vi "Generate PCB coverage.vi"(0 "Inspection Data":T2, 5 "error in (no error)":errorcluster) -> (12 "DataOut":T1, 19 "error out":errorcluster)   [LabVIEW 2013, in "Manipulate IPF.lvlib"]
uses:
  Manipulate IPF.lvlib
  3013/code/Modules/GUI/GUI_5/subPanels/edit/type_def/data.ctl
  3013/code/Modules/Configuration/type_def/Scan Params.ctl
  3013/code/Modules/Configuration/type_def/Profile Resolution.ctl
  3013/code/Modules/Preprocess Data/type_def/direction.ctl
  3013/code/Modules/Inspection/Data/Panel_class/type_def/Config File data.ctl
  3013/code/Modules/Inspection/type_def/Pos and Rot.ctl
  3013/code/Modules/Inspection/Data/PCB_class/type_def/PCB Params.ctl
  3013/code/Modules/Inspection/Data/Panel_class/type_def/BarCode Params.ctl
  3013/code/Modules/Barcode Reader/type_def/id.ctl
  3013/code/Modules/Inspection/Data/Panel_class/type_def/inspection data.ctl
  3013/code/Modules/Inspection/type_def/Range Limits.ctl
  <userlib>/_OpenG.lib/file/file.llb/File Exists - Scalar__ogtk.vi
  <vilib>/Utility/file.llb/Read From Spreadsheet File (string).vi
  <userlib>/_OpenG.lib/file/file.llb/Convert File Extension (String)__ogtk.vi
  <vilib>/Utility/file.llb/Write To Spreadsheet File (string).vi
  <userlib>/_OpenG.lib/string/string.llb/Trim Whitespace (String)__ogtk.vi
  <vilib>/Utility/file.llb/Read From Spreadsheet File (DBL).vi
  Mike/APG_mike a3Di.lvlib
  3D Viewer/3D Viewer.lvlib
  <vilib>/Analysis/geometry.llb/Point in Polygon Position.ctl
  <vilib>/Analysis/NI_AAL_Geometry.lvlib
  <vilib>/Analysis/geometry.llb/Point in Polygon (Array).vi
  3013/code/subVIs/Library/array/AmFax Array.lvlib
  3013/code/Modules/Inspection/Inspection.lvlib
  3013/code/Modules/Inspection/Data/PCB_class/PCB.lvclass
  3013/code/Modules/Barcode Reader/Barcode Reader.lvlib
  3013/code/Modules/Inspection/Data/Panel_class/Panel.lvclass
  3013/code/Modules/Configuration/Config.lvlib
  3013/code/Modules/Preprocess Data/PreProcess.lvlib
  3013/code/Modules/GUI/GUI_5/subPanels/edit/edit.lvlib
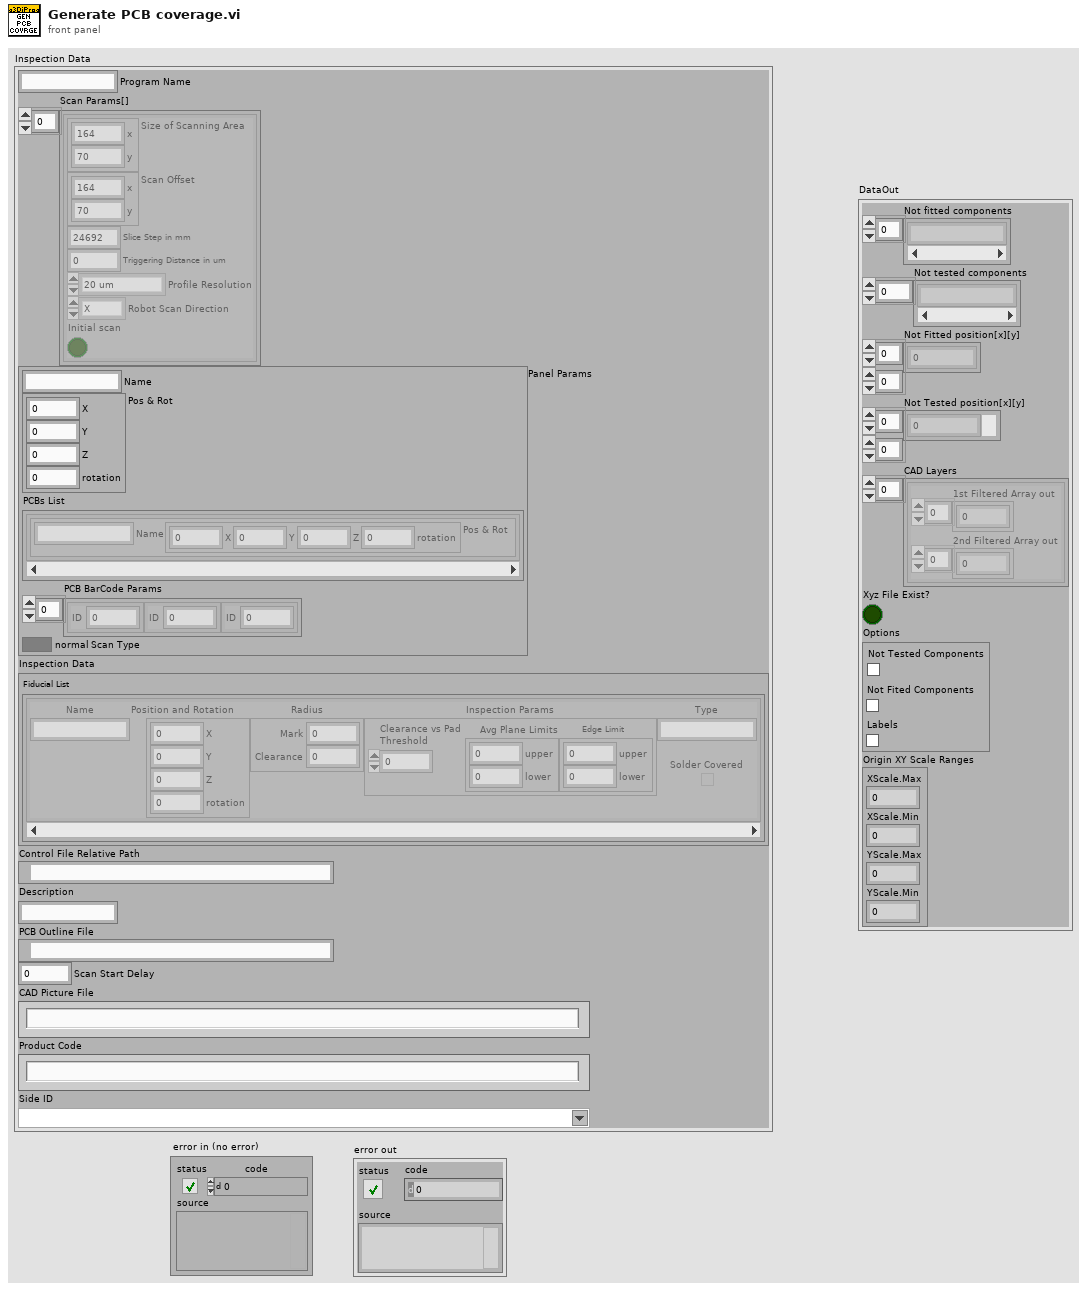
[diagram p1: front panel]
types:
  T1 = cluster{"Not fitted components":string[], "Not tested components":string[], "Not Fitted position[x][y] ":dbl[][], "Not Tested position[x][y]":dbl[][], "CAD Layers":cluster{"1st Filtered Array out":sgl[], "2nd Filtered Array out":sgl[]}[], "Xyz File Exist? ":bool, "Options":cluster{"Enable Not Tested Components":bool, "Enable Not Fited Components":bool, "Enable Labels":bool}, "Origin XY Scale Ranges":cluster{"XScale.Max":dbl, "XScale.Min":dbl, "YScale.Max":dbl, "YScale.Min":dbl}}
  T2 = typedef "GUI.lvlib/subPanel.lvlib/edit.lvlib/data.ctl" = cluster{"Program Name":string, "Scan Params[]":T3[], "Panel Params":T6, "Inspection Data":T11, "Control File Relative Path":path, "Description":string, "PCB Outline File":path, "Scan Start Delay":dbl, "CAD Picture File":string, "Product Code":string, "Side ID":string}
  T3 = typedef "Config.lvlib/Scan Params.ctl" = cluster{"Size of Scanning Area":cluster{"x":dbl, "y":dbl}, "Scan Offset":cluster{"x":dbl, "y":dbl}, "Slice Step in mm":dbl, "Triggering Distance in mm":dbl, "Triggering Distance in um":dbl, "Profile Resolution":T4, "Version":string, "Robot Scan Direction":T5, "Initial scan":bool}
  T4 = typedef "Config.lvlib/Profile Resolution.ctl" = enum8{"20 um", "40 um"}
  T5 = typedef "PreProcess.lvlib/direction.ctl" = enum8{"X", "Y"}
  T6 = typedef "Inspection.lvlib/Panel.lvclass/Config File data.ctl" = cluster{"Name":string, "Pos & Rot":T7, "PCBs List":cluster{"PCB Params":T8}[], "PCB BarCode Params":T9[], "Scan Type":bool}
  T7 = typedef "Inspection.lvlib/Pos and Rot.ctl" = cluster{"X":dbl, "Y":dbl, "Z":dbl, "rotation":dbl}
  T8 = typedef "Inspection.lvlib/PCB.lvclass/PCB Params.ctl" = cluster{"Name":string, "Pos & Rot":T7}
  T9 = typedef "Inspection.lvlib/Panel.lvclass/BarCode Params.ctl" = cluster{"ID":T10}
  T10 = typedef "Barcode Reader.lvlib/id.ctl" = u8
  T11 = typedef "Inspection.lvlib/Panel.lvclass/inspection data.ctl" = cluster{"Fiducial List":cluster{"Name":string, "Position and Rotation":T7, "Radius":cluster{"Mark":dbl, "Clearance":dbl}, "Inspection Params":cluster{"Clearance vs Pad\nThreshold":dbl, "Avg Plane Limits":T12, "Edge Limit":T12}, "Type":string, "Solder Covered":bool}[]}
  T12 = typedef "Inspection.lvlib/Range Limits.ctl" = cluster{"upper":sgl, "lower":sgl}
  T13 = cluster{"ODB2CPF.exe":path, "TCFToArtworkCPF.exe":path, "TCFToCPFLabels.exe":path, "7z.exe":path, "UpdateTCFLibrary.exe":path, "a3DiPackageTests":path, "Error Codes":path, "TCFToCuboidRefCPF":path, "TCFToArtworkRefCPF":path, "ExtractPKG":path, "ExtractTCFFromODBFileForPKG":path, "OutLineFilterTCFPKG":path, "GenerateLibraryFromTCF":path, "FlipCPF":path, "FlipTCF":path, "TCFToJointBridgeCPF":path, "TCFToJointFR4CPF":path, "UpdateTCFPartNoFrCompName":path}
  T14 = typedef "NI_AAL_Geometry.lvlib/Point in Polygon Position.ctl" = u16
  T15 = cluster{"1st Filtered Array out":sgl[], "2nd Filtered Array out":sgl[]}
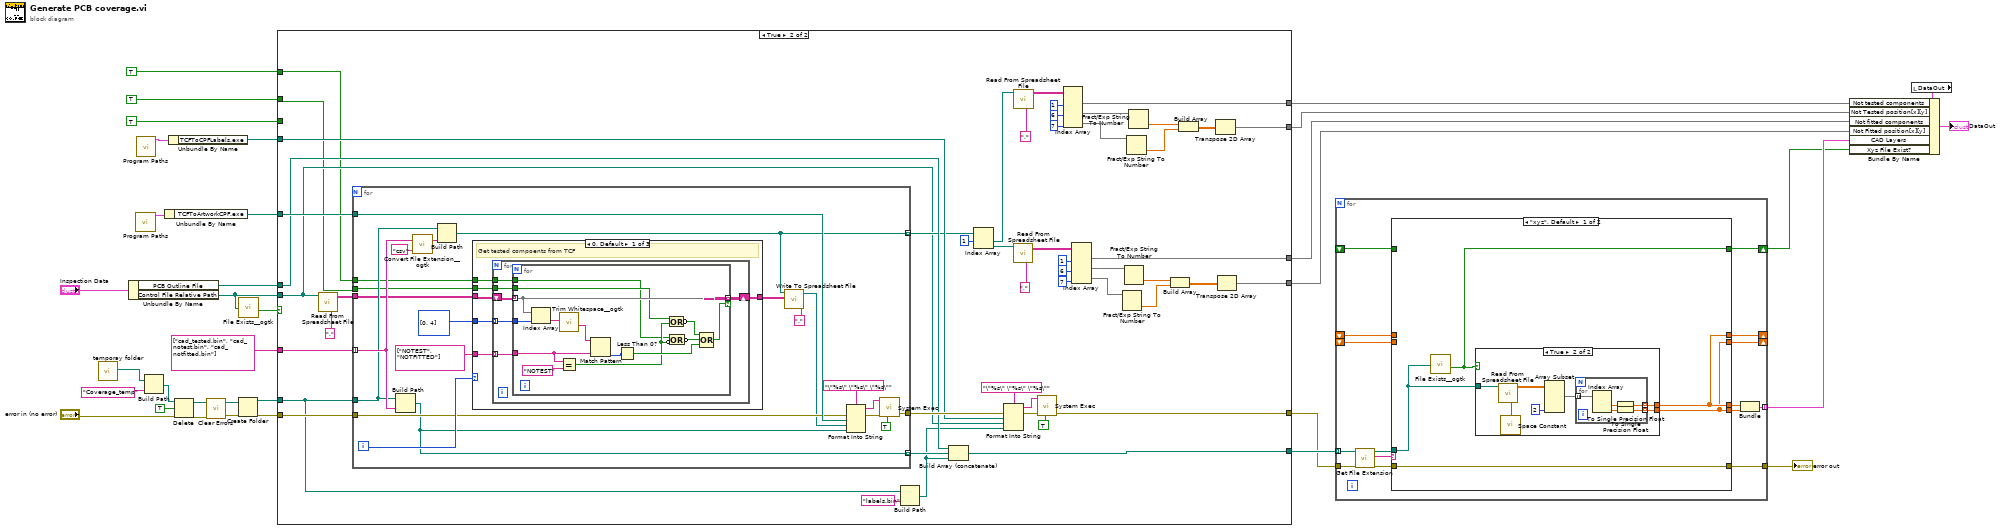
[diagram p0: block diagram]
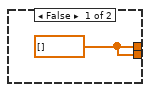
[diagram p2: hidden frame]
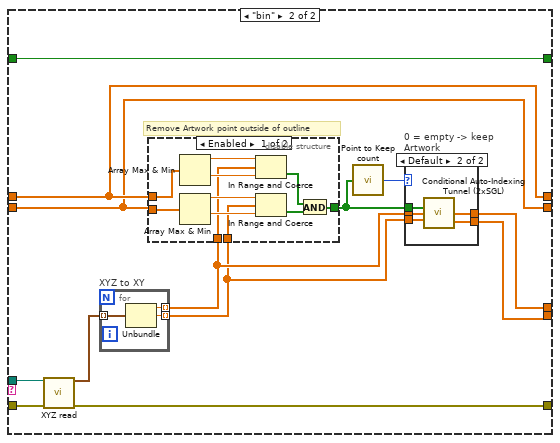
[diagram p3: hidden frame]
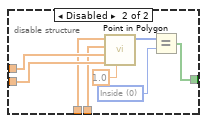
[diagram p5: hidden frame]
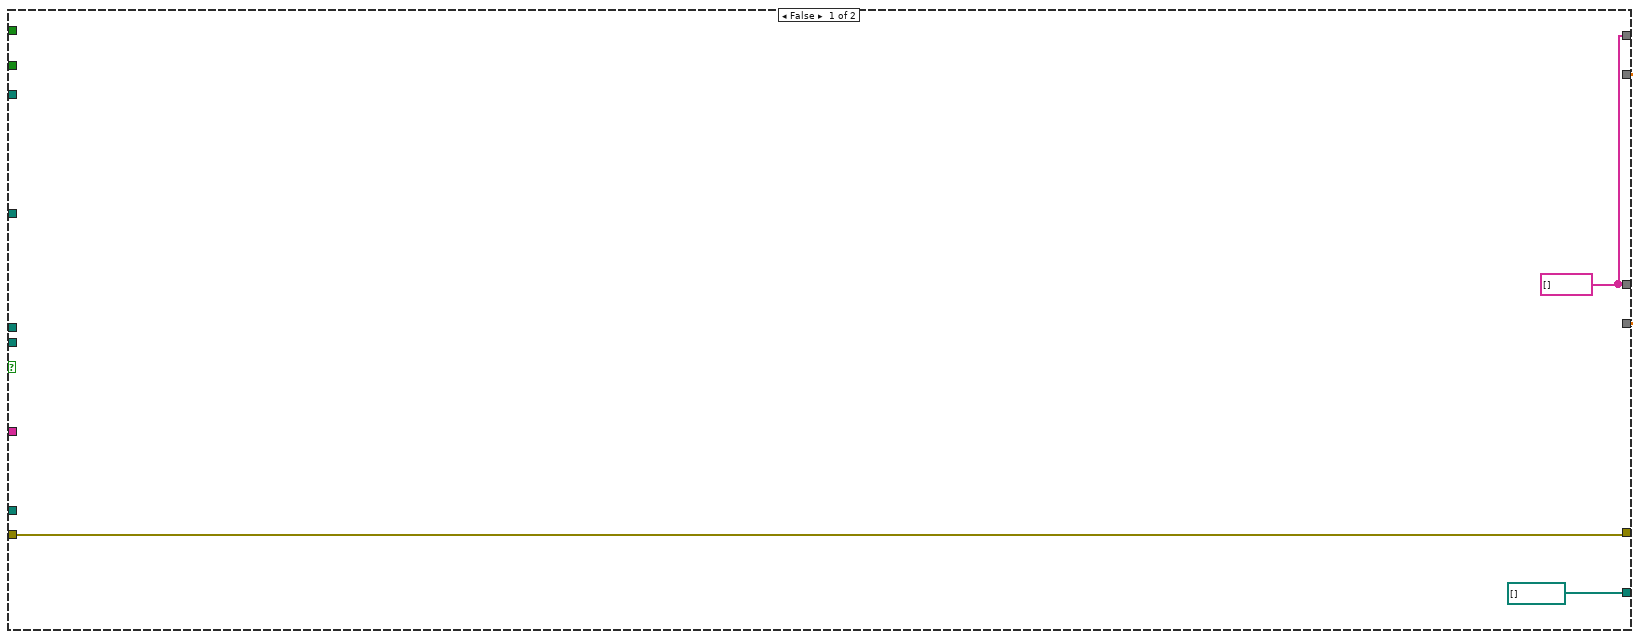
[diagram p6: hidden frame]
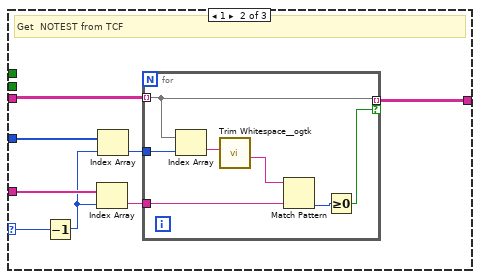
[diagram p7: hidden frame]
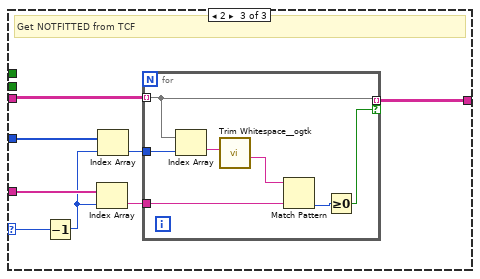
[diagram p8: hidden frame]
diagram:
  n1 = call "temporay folder.vi"() -> ("temporay folder"=w33:path)  [unwired: 11 in]
  n2 = Unbundle By Name("Inspection Data") -> ("PCB Outline File"=w15:path, "Control File Relative Path"=w17:path)
  n3 = call "Program Paths.vi"() -> ("Program paths"=w31:T13)  [unwired: 10 in]
  n4 = call "Program Paths.vi"() -> ("Program paths"=w21:T13)  [unwired: 10 in]
  n5 = Build Path(base path=w33, name or relative path="Coverage_temp") -> (appended path=w27:path)
  n6 = Unbundle By Name(w31) -> ("TCFToArtworkCPF.exe"=w28:path)
  n7 = Unbundle By Name(w21) -> ("TCFToCPFLabels.exe"=w20:path)
  n8 = Delete(path (use dialog)=w27, entire hierarchy (F)=TRUE, error in="error in (no error)") -> (deleted path=w23:path, error out=w25:errorcluster)  [unwired: 2 in, 1 out]
  n9 = call <vilib>:"Clear Errors.vi"("error in (no error)"=w25) -> ("error out"=w24:errorcluster)  [unwired: 6 in]
  n10 = Create Folder(path (use dialog)=w23, error in=w24) -> (created path=w19:path, error out=w22:errorcluster)  [unwired: 1 in, 1 out]
  n11 = call-poly <userlib>:"File Exists__ogtk.vi"("file path"=w17) -> ("exists"=w16:bool)  [unwired: 6 in, 1 out]
  n12 = case shown="True" w16 {
    tunnel: string[] ["cad_tested.bin", "cad_notest.bin", "cad_notfitted.bin"] -> [_ w87]
    tunnel: w28 -> [_ w86]
    tunnel: w22 -> [w38 w85]
    tunnel: [w38 w83] -> w2
    tunnel: w20 -> [_ w82]
    tunnel: w19 -> [_ w81]
    tunnel: w17 -> [_ w48]
    tunnel: w15 -> [_ w78]
    tunnel: [w37 w70] -> w11
    tunnel: [w37 w62] -> w14
    tunnel: [dbl[][] [] w50] -> w9
    tunnel: [dbl[][] [] w52] -> w10
    tunnel: TRUE ("Not Fited Components") -> [_ w46]
    tunnel: TRUE ("Not Tested Components") -> [_ w45]
    tunnel: TRUE ("Labels") -> [_ _]
    tunnel: [path[] [] w44] -> w5
    frame False {
      w37 = string[] [] ("all rows")
    }
    frame True {
      n13 = call-poly <vilib>:"Read From Spreadsheet File.vi"("delimiter (\\t)"="," ("delimiter (\\t)"), "file path (dialog if empty)"=w48) -> ("all rows"=w47:string[][])  [unwired: 5 in, 4 out]
      n14 = for {
        tunnel: w87 -> [w103] mode=indexing
        tunnel: w85 -> [w99]
        tunnel: w81 -> [w102]
        tunnel: w86 -> [w101]
        tunnel: [w98] -> w84
        tunnel: [w88] -> w79 mode=indexing
        tunnel: [w92] -> w77 mode=indexing
        tunnel: w47 -> [w91]
        tunnel: w46 -> [w90]
        tunnel: w45 -> [w89]
        i -> [w100]
        n15 = Build Path(base path=w102, name or relative path=w103) -> (appended path=w88:path)
        n16 = call-poly <userlib>:"Convert File Extension__ogtk.vi"("new ending (none)"="csv", "file name"=w103) -> ("new filename"=w109:string)  [unwired: 1 out]
        n17 = Build Path(base path=w102, name or relative path=w109) -> (appended path=w92:path)
        n18 = case shown="0, Default" w100 {
          selector: w100 -> [_ w143 w158]
          tunnel: w91 -> [w115 w142 w157]
          tunnel: [w114 w141 w156] -> w95
          tunnel: i32[] [0, 4] -> [w113 w140 w155]
          tunnel: string[] ["NOTEST", "NOTFITTED"] -> [w112 w139 w154]
          tunnel: w90 -> [w110 _ _]
          tunnel: w89 -> [w111 _ _]
          frame 0, Default {
            # "Get tested compoents from TCF"
            n19 = for {
              tunnel: w113 -> [w119] mode=indexing
              tunnel: w112 -> [w120] mode=indexing
              shift-right: [w121] -> w114
              shift-left: w115 -> [w118]
              tunnel: w111 -> [w116]
              tunnel: w110 -> [w117]
              n20 = for {
                tunnel: w118 -> [w135] mode=indexing
                tunnel: [w135] -> w121 mode=indexing if=w130
                tunnel: w120 -> [w128]
                tunnel: w119 -> [w131]
                tunnel: w117 -> [w123]
                tunnel: w116 -> [w122]
                n21 = Index Array(array=w135, index=w131) -> (element=w134:string)
                n22 = call-poly <userlib>:"Trim Whitespace__ogtk.vi"("String in"=w134) -> ("String out"=w133:string)  [unwired: 6 in]
                n23 = Equal?(x=w128, y="NOTEST") -> (x = y?=w125:bool)
                n24 = Match Pattern(string=w133, regular expression=w128) -> (offset past match=w132:i32)  [unwired: 1 in, 3 out]
                n25 = Less Than 0?(x=w132) -> (x < 0?=w126:bool)
                n26 = Compound Arithmetic op=OR(w123, w125) -> (invert w124:bool)
                n27 = Compound Arithmetic op=OR(w122, invert w125) -> (invert w129:bool)
                n28 = Compound Arithmetic op=OR(w124, w129, w126) -> (w130:bool)
              }
            }
          }
          frame 1 {
            # "Get  NOTEST from TCF"
            n29 = Decrement(x=w143) -> (x-1=w136:i32)
            n30 = Index Array(array=w139, index=w136) -> (element=w138:string)
            n31 = Index Array(array=w140, index=w136) -> (element=w137:i32)
            n32 = for {
              tunnel: w142 -> [w150] mode=indexing
              tunnel: [w150] -> w141 mode=indexing if=w146
              tunnel: w138 -> [w145]
              tunnel: w137 -> [w144]
              n33 = Index Array(array=w150, index=w144) -> (element=w149:string)
              n34 = call-poly <userlib>:"Trim Whitespace__ogtk.vi"("String in"=w149) -> ("String out"=w148:string)  [unwired: 6 in]
              n35 = Match Pattern(string=w148, regular expression=w145) -> (offset past match=w147:i32)  [unwired: 1 in, 3 out]
              n36 = Greater Or Equal To 0?(x=w147) -> (x >= 0?=w146:bool)
            }
          }
          frame 2 {
            # "Get NOTFITTED from TCF"
            n37 = Decrement(x=w158) -> (x-1=w151:i32)
            n38 = Index Array(array=w154, index=w151) -> (element=w153:string)
            n39 = Index Array(array=w155, index=w151) -> (element=w152:i32)
            n40 = for {
              tunnel: w157 -> [w165] mode=indexing
              tunnel: [w165] -> w156 mode=indexing if=w161
              tunnel: w153 -> [w160]
              tunnel: w152 -> [w159]
              n41 = Index Array(array=w165, index=w159) -> (element=w164:string)
              n42 = call-poly <userlib>:"Trim Whitespace__ogtk.vi"("String in"=w164) -> ("String out"=w163:string)  [unwired: 6 in]
              n43 = Match Pattern(string=w163, regular expression=w160) -> (offset past match=w162:i32)  [unwired: 1 in, 3 out]
              n44 = Greater Or Equal To 0?(x=w162) -> (x >= 0?=w161:bool)
            }
          }
        }
        n45 = call-poly <vilib>:"Write To Spreadsheet File.vi"("delimiter (\\t)"="," ("delimiter (\\t)"), "2D data"=w95, "file path (dialog if empty)"=w92) -> ("new file path (Not A Path if cancelled)"=w96:path)  [unwired: 5 in]
        n46 = Format Into String(format string="\"%s\" \"%s\" \"%s\"", error in=w99, w101, w96, w88) -> (resulting string=w104:string, error out=w106:errorcluster)  [unwired: 1 in]
        n47 = call <vilib>:"System Exec.vi"("run minimized? (F)"=TRUE, "error in (no error)"=w106, "command line"=w104) -> ("error out"=w98:errorcluster)  [unwired: 5 in, 3 out]
      }
      n48 = Build Path(base path=w81, name or relative path="labels.bin") -> (appended path=w39:path)
      n49 = Build Array (concatenate)(w78, w79, w39) -> (w44:path[])
      n50 = Index Array(array=w77, index #1=1 ("index")) -> (element #1=w73:path, element #2=w71:path)  [unwired: 1 in]
      n51 = Format Into String(format string="\"%s\" \"%s\" \"%s\"", error in=w84, w82, w48, w39) -> (resulting string=w43:string, error out=w41:errorcluster)  [unwired: 1 in]
      n52 = call-poly <vilib>:"Read From Spreadsheet File.vi"("delimiter (\\t)"="," ("delimiter (\\t)"), "file path (dialog if empty)"=w71) -> ("all rows"=w63:string[][])  [unwired: 5 in, 4 out]
      n53 = call-poly <vilib>:"Read From Spreadsheet File.vi"("delimiter (\\t)"="," ("delimiter (\\t)"), "file path (dialog if empty)"=w73) -> ("all rows"=w75:string[][])  [unwired: 5 in, 4 out]
      n54 = call <vilib>:"System Exec.vi"("run minimized? (F)"=TRUE, "error in (no error)"=w41, "command line"=w43) -> ("error out"=w83:errorcluster)  [unwired: 5 in, 3 out]
      n55 = Index Array(array=w75, index (col) #1=1 ("disabled index (col)"), index (col) #2=6 ("index (col)"), index (col) #3=7 ("index (col)")) -> (element #1=w70:string[], element #2=w55:string[], element #3=w54:string[])  [unwired: 3 in]
      n56 = Index Array(array=w63, index (col) #1=1 ("disabled index (col)"), index (col) #2=6 ("index (col)"), index (col) #3=7 ("index (col)")) -> (element #1=w62:string[], element #2=w61:string[], element #3=w60:string[])  [unwired: 3 in]
      n57 = Fract/Exp String To Number(string=w60) -> (number=w58:dbl[])  [unwired: 3 in, 1 out]
      n58 = Fract/Exp String To Number(string=w61) -> (number=w59:dbl[])  [unwired: 3 in, 1 out]
      n59 = Fract/Exp String To Number(string=w54) -> (number=w57:dbl[])  [unwired: 3 in, 1 out]
      n60 = Fract/Exp String To Number(string=w55) -> (number=w56:dbl[])  [unwired: 3 in, 1 out]
      n61 = Build Array(w59, w58) -> (w51:dbl[][])
      n62 = Build Array(w56, w57) -> (w53:dbl[][])
      n63 = Transpose 2D Array(2D array=w53) -> (transposed array=w52:dbl[][])
      n64 = Transpose 2D Array(2D array=w51) -> (transposed array=w50:dbl[][])
    }
  }
  n65 = for {
    tunnel: [w180] -> w4
    tunnel: [w179] -> w3 mode=indexing
    shift-right: [w174] -> _
    shift-left: _ -> [w172]
    shift-right: [w171] -> _
    shift-left: _ -> [w173]
    shift-right: [w170] -> w1
    shift-left: _ -> [w169]
    tunnel: w5 -> [w167] mode=indexing
    tunnel: w2 -> [w166]
    n66 = call <vilib>:"Get File Extension.vi"("error in (no error)"=w166, "file"=w167) -> ("error out"=w178:errorcluster, "lowercase file extension"=w176:string, "dup file"=w177:path)  [unwired: 6 in, 1 out]
    n67 = case shown="\"xyz\", Default" w176 {
      tunnel: w177 -> [w182 w211]
      tunnel: w178 -> [w185 w210]
      tunnel: [w185 w209] -> w180
      tunnel: [w184 w204] -> w168
      tunnel: [w183 w205] -> w175
      tunnel: [w184 w203] -> w174
      tunnel: w173 -> [_ w202]
      tunnel: w172 -> [_ w203]
      tunnel: [w183 w202] -> w171
      tunnel: [w181 w199] -> w170
      tunnel: w169 -> [_ w199]
      frame "xyz", Default {
        n68 = call-poly <userlib>:"File Exists__ogtk.vi"("file path"=w182) -> ("exists"=w181:bool)  [unwired: 6 in, 1 out]
        n69 = case shown="True" w181 {
          tunnel: [w186 w189] -> w184
          tunnel: [w186 w188] -> w183
          tunnel: w182 -> [_ w187]
          frame False {
            w186 = sgl[] []
          }
          frame True {
            n70 = call <vilib>:"Space Constant.vi"() -> ("String"=w191:string)
            n71 = call-poly <vilib>:"Read From Spreadsheet File.vi"("delimiter (\\t)"=w191, "file path (dialog if empty)"=w187) -> ("all rows"=w193:dbl[][])  [unwired: 5 in, 4 out]
            n72 = Array Subset(array=w193, length (col)=2 ("length")) -> (w190:dbl[][])  [unwired: 3 in]
            n73 = for {
              tunnel: w190 -> [w198] mode=indexing
              tunnel: [w194] -> w189 mode=indexing
              tunnel: [w195] -> w188 mode=indexing
              n74 = Index Array(array=w198) -> (element #1=w197:dbl, element #2=w196:dbl)  [unwired: 2 in]
              n75 = To Single Precision Float(number=w197) -> (single precision float=w194:sgl)
              n76 = To Single Precision Float(number=w196) -> (single precision float=w195:sgl)
            }
          }
        }
      }
      frame "bin" {
        # "Remove Artwork point outside of outline"
        n77 = call "XYZ read.vi"("XYZ file"=w211, "error in (no error)"=w210) -> ("Position[]"=w208:cluster{"X":sgl, "Y":sgl, "Z":sgl}[], "error out"=w209:errorcluster)  [unwired: 11 in, 1 out]
        n78 = for "XYZ to XY" {
          tunnel: w208 -> [w240] mode=indexing
          tunnel: [w239] -> w201 mode=indexing
          tunnel: [w238] -> w200 mode=indexing
          n79 = Unbundle(w240) -> ("X"=w239:sgl, "Y"=w238:sgl)  [unwired: 1 out]
        }
        n80 = disable-structure shown="Enabled" {
          disable-tunnel: w202 -> [w223 w232]
          disable-tunnel: w201 -> [w222 w230]
          disable-tunnel: w200 -> [w221 w231]
          disable-tunnel: [w220 w234] -> w207
          disable-tunnel: w203 -> [w219 w233]
          frame Enabled {
            n81 = Array Max & Min(array=w219) -> (max value=w229:sgl, min value=w228:sgl)  [unwired: 2 out]
            n82 = Array Max & Min(array=w223) -> (max value=w226:sgl, min value=w227:sgl)  [unwired: 2 out]
            n83 = In Range and Coerce(upper limit=w229, x=w222, lower limit=w228) -> (In Range?=w225:bool[])  [unwired: 1 out]
            n84 = In Range and Coerce(upper limit=w226, x=w221, lower limit=w227) -> (In Range?=w224:bool[])  [unwired: 1 out]
            n85 = And(x=w225, y=w224) -> (x .and. y?=w220:bool[])
          }
          frame Disabled {
            w236 = T14 0 items=["Inside", "On Boundary", "Outside"] ("position")
            n86 = call-poly <vilib>:"Point in Polygon.vi"("tolerance"=1.0, "Polygon Y"=w232, "Polygon X"=w233, "Y"=w231, "X"=w230) -> ("Position"=w235:T14[])  [unwired: 5 in, 1 out]
            n87 = Equal?(x=w235, y=w236) -> (x = y?=w234:bool[])
          }
        }
        n88 = call "Point to Keep count.vi"("Points to keep[]"=w207) -> ("TRUEs count"=w206:i32)  [unwired: 14 in]
        n89 = case "0 = empty -> keep Artwork" shown="Default" w206 {
          tunnel: [w213 w218] -> w204
          tunnel: [w212 w217] -> w205
          tunnel: w201 -> [w213 w216]
          tunnel: w200 -> [w212 w215]
          tunnel: w207 -> [_ w214]
          frame 0 {
          }
          frame Default {
            n90 = call "Conditional Auto-Indexing Tunnel (2xSGL).vi"("Elements to keep"=w214, "1st Array in"=w216, "2nd Array in"=w215) -> ("1st Filtered Array out"=w218:sgl[], "2nd Filtered Array out"=w217:sgl[])  [unwired: 11 in]
          }
        }
      }
    }
    n91 = Bundle("1st Filtered Array out"=w168, "2nd Filtered Array out"=w175) -> (w179:T15)  [unwired: 1 in]
  }
  "error out" <- w4
  n92 = local read "DataOut"() -> (w7:T1)
  n93 = Bundle By Name(cluster=w7, "Not tested components"=w11, "Not Tested position[x][y]"=w10, "Not fitted components"=w14, "Not Fitted position[x][y]"=w9, "CAD Layers"=w3, "Xyz File Exist?"=w1) -> (→"DataOut":T1)
